vi "Remove Header.vi"(8 "error in":errorcluster, 10 "header":T1, 11 "session in":refnum<class "Session.lvclass">) -> (0 "error out":errorcluster, 3 "session out":refnum<class "Session.lvclass">)   [LabVIEW 2019, in "NI_Advanced HTTP Client.lvlib" / "Session.lvclass"]
doc: "Removes a header field line from all web requests associated with the HTTP session. Headers define attributes of the data exchanged between the client and server."
uses:
  Session.lvclass
  Header--Combo Box.ctl
  Session.lvclass/Session.ctl
  lvwebclient_64.dll
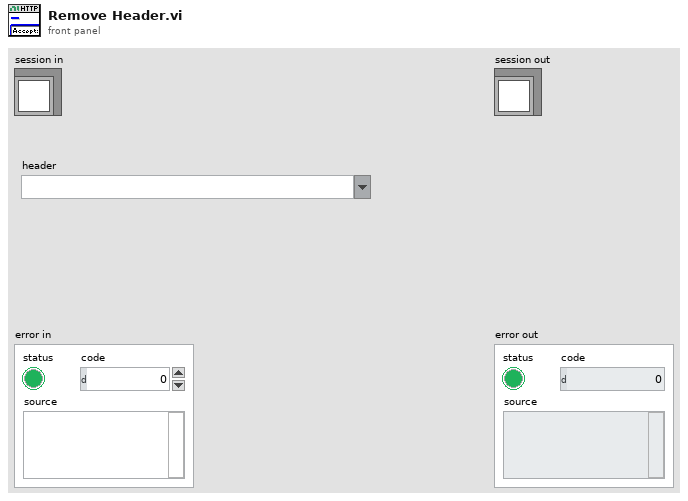
[diagram p1: front panel]
types:
  T1 = typedef "NI_Advanced HTTP Client.lvlib/Session.lvclass/Header--Combo Box.ctl" = string
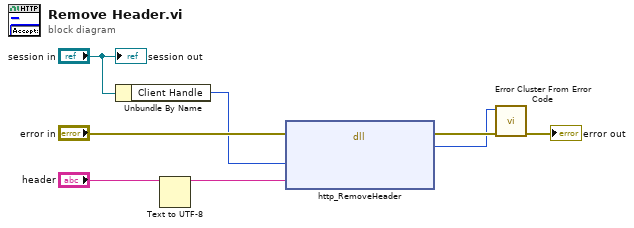
[diagram p0: block diagram]
diagram:
  n1 = Unbundle By Name("session in") -> ("Client Handle"=w2:u32)
  n2 = Text to UTF-8(11:"header") -> (3:w1:string)  [unwired: 2 in, 1 out]
  n3 = dll-call lib="C:/Users/Localization Tester/Desktop/Advanced HTTP Client/lvwebclient_*.*" fn="http_RemoveHeader"(error in="error in", "handle"=w2, "headerName"=w1) -> (error out=w4:errorcluster, "return"=w3:i32)  [unwired: 4 in, 1 out]
  n4 = call <vilib>:"Error Cluster From Error Code.vi"("error in (no error)"=w4, "error code (0)"=w3) -> ("error out"=→"error out":errorcluster)  [unwired: 7 in]
  "session out" <- "session in"
